vi "Get Advanced System Info - Example.vi"() -> ()   [LabVIEW 2015, in "SMI.lvlib"]
uses:
  SMI.lvlib
  <vilib>/nisyscfg/Close (Hardware).vi
  classes/SysCfg Device/SysCfg Device.lvclass
  classes/Controller/Controller.lvclass
  <resource>/objmgr/nisysapi.rc
  <resource>/objmgr/niflexriosae.rc
  <vilib>/nisyscfg/nisyscfg.lvlib
panel:
  in  "NI Auth":cluster{"User Name":string, "Password":string}[](array[cluster])
  out "error out":errorcluster
  out "Startup Settings:Disable RT Startup App":bool
  out "Real-Time:System Status":string
  out "Operating System:Architecture":string
  in  "Target Address":string
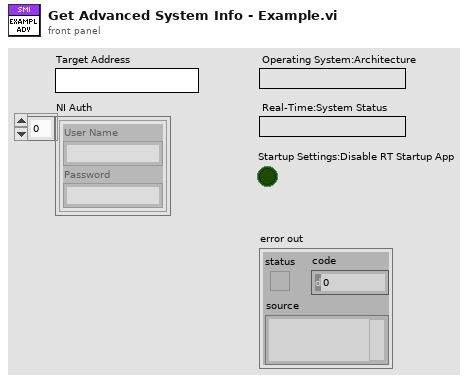
[diagram p1: front panel]
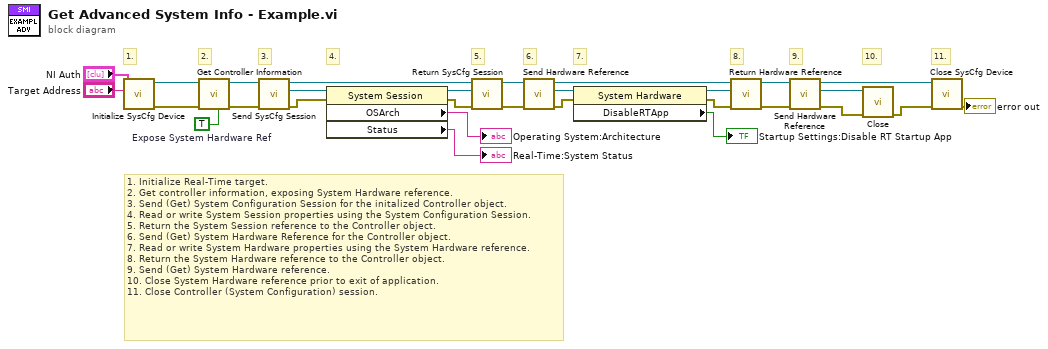
[diagram p0: block diagram]
diagram:
  w25 = TRUE  # Expose System Hardware Ref
  # "11."
  # "10."
  # "9."
  # "8."
  # "7."
  # "6."
  # "5."
  # "4."
  # "3."
  # "2."
  # "1."
  # "1. Initialize Real-Time target.\n2. Get controller information, exposing System Hardware reference.\n3. Send (Get) System Configuration Session for the initalized Controller object.\n4. Read or write System Session properties using the System Configuration Session.\n5. Return the System Session reference to the Controller object.\n6. Send (Get) System Hardware Reference for the Controller object.\n7. Read or write System Hardware properties using the System Hardware reference.\n8. Return the System Hardware reference to the Controller object.\n9. Send (Get) System Hardware reference.\n10. Close System Hardware reference prior to exit of application.\n11. Close Controller (System Configuration) session."
  n1 = call "Initialize SysCfg Device.vi"("NI Auth"="NI Auth", "Target Address"="Target Address") -> ("error out"=w29:errorcluster, "Controller out"=w27:refnum<class "Controller.lvclass">)  [unwired: 8 in]
  n2 = call "Get Controller Information.vi"("Expose System Hardware Reference (F)"=w25, "error in"=w29, "Controller in"=w27) -> ("error out"=w26:errorcluster, "Controller out"=w28:refnum<class "Controller.lvclass">)  [unwired: 6 in, 1 out]
  n3 = call "Send SysCfg Session.vi"("error in"=w26, "Controller in"=w28) -> ("error out"=w23:errorcluster, "SysCfg Session"=w24:refnum<k21>, "Controller out"=w20:refnum<class "Controller.lvclass">)  [unwired: 7 in]
  n4 = property class="System Session"(reference=w24, error in=w23) -> (reference out=w21:refnum<k21>, error out=w22:errorcluster, "OSArch"=→"Operating System:Architecture":string, "Status"=→"Real-Time:System Status":string)
  n5 = call "Return SysCfg Session.vi"("error in"=w22, "SysCfg Session"=w21, "Controller in"=w20) -> ("error out"=w18:errorcluster, "Controller out"=w19:refnum<class "Controller.lvclass">)  [unwired: 7 in]
  n6 = call "Send Hardware Reference.vi"("error in"=w18, "Controller in"=w19) -> ("error out"=w15:errorcluster, "System Hardware Reference"=w17:refnum<k20>, "Controller out"=w13:refnum<class "Controller.lvclass">)  [unwired: 7 in]
  n7 = property class="System Hardware"(reference=w17, error in=w15) -> (reference out=w16:refnum<k20>, error out=w14:errorcluster, "DisableRTApp"=→"Startup Settings:Disable RT Startup App":bool)
  n8 = call "Return Hardware Reference.vi"("error in"=w14, "System Hardware Reference"=w16, "Controller in"=w13) -> ("error out"=w10:errorcluster, "Controller out"=w9:refnum<class "Controller.lvclass">)  [unwired: 7 in]
  n9 = call "Send Hardware Reference.vi"("error in"=w10, "Controller in"=w9) -> ("error out"=w12:errorcluster, "System Hardware Reference"=w11:refnum<k20>, "Controller out"=w7:refnum<class "Controller.lvclass">)  [unwired: 7 in]
  n10 = call-poly <vilib>:"Close.vi"("error in (no error)"=w12, "Resource in"=w11) -> ("error out"=w8:errorcluster)  [unwired: 9 in]
  n11 = call "Close SysCfg Device.vi"("error in"=w8, "Controller in"=w7) -> ("error out"=→"error out":errorcluster)  [unwired: 9 in]
